vi "Set LED Mode.vi"(8 "error in (no error)":errorcluster, 10 "Numeric":dbl, 11 "SerialPortRef":T1) -> (0 "error out":errorcluster, 3 "SerialPortRef 2":T1)   [LabVIEW 2015]
uses:
  <vilib>/Rock Robotics/WPI/SerialPort/WPI_SerialPortRef.ctl
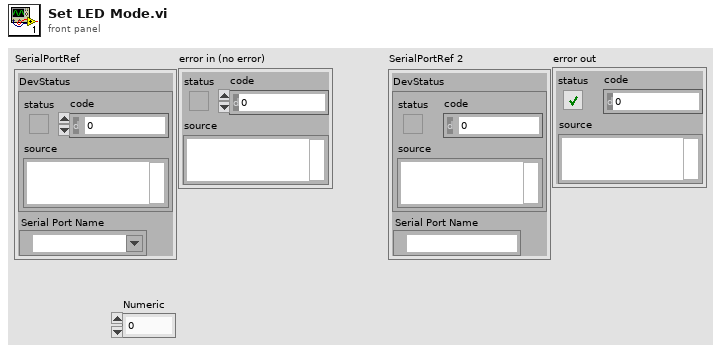
[diagram p1: front panel]
types:
  T1 = typedef "WPI_SerialPortRef.ctl" = cluster{"DevStatus":errorcluster, "Serial Port Name":refnum<visa-resource-name>}
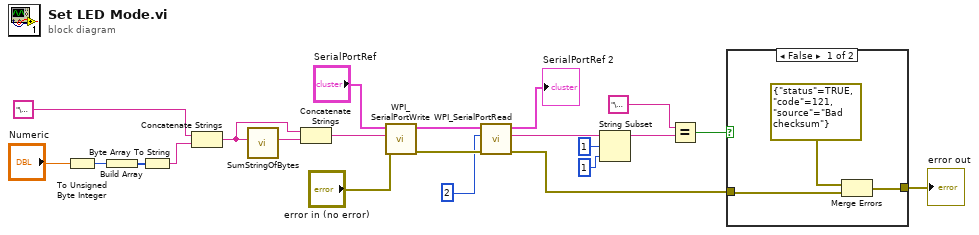
[diagram p0: block diagram]
diagram:
  n1 = To Unsigned Byte Integer(number="Numeric") -> (unsigned 8bit integer=w19:u8)
  n2 = Build Array(w19) -> (w18:u8[])
  n3 = Byte Array To String(unsigned byte array=w18) -> (string=w16:string)
  n4 = Concatenate Strings("\u0014", w16) -> (w14:string)
  n5 = call "SumStringOfBytes.vi"("String Of Bytes"=w14) -> ("SumAsString"=w13:string)  [unwired: 10 in]
  n6 = Concatenate Strings(w14, w13) -> (w12:string)
  n7 = call <vilib>:"WPI_SerialPortWrite.vi"("error in (no error)"="error in (no error)", "Buffer"=w12, "SerialPortRef"="SerialPortRef") -> ("error out"=w22:errorcluster, "SerialPortRef"=w2:T1)  [unwired: 6 in, 1 out]
  n8 = call <vilib>:"WPI_SerialPortRead.vi"("error in (no error)"=w22, "Num Bytes to Read"=2, "SerialPortRef"=w2) -> ("error out"=w5:errorcluster, "Buffer"=w11:string, "SerialPortRef"=→"SerialPortRef 2":T1)  [unwired: 6 in]
  n9 = String Subset(string=w11, offset (0)=1, length (rest)=1 ("length (rest)")) -> (substring=w8:string)
  n10 = Equal?(x="\u0014", y=w8) -> (x = y?=w6:bool)
  n11 = case shown="False" w6 {
    tunnel: w5 -> [w24 w26]
    tunnel: [w23 w26] -> w4
    frame False {
      n12 = Merge Errors(errorcluster {"status"=TRUE, "code"=121, "source"="Bad checksum"} ("error in"), w24) -> (w23:errorcluster)
    }
    frame True {
    }
  }
  "error out" <- w4
